vi "Get VS Amplitude String.vi"(10 "text":string, 11 "index":i32) -> (2 "text out":string, 3 "function return":u32)   [LabVIEW 2018, in "Copy of Andor SDK.lvlib"]
doc: "EXPNETTYPE unsigned int WINAPI GetVSAmplitudeString(int index, char * text);"
uses:
  Copy of Andor SDK.lvlib
  <userlib>/Andor SDK/ATMCD32D.dll
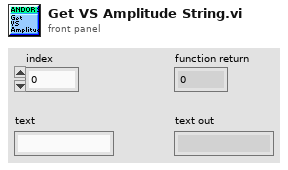
[diagram p1: front panel]
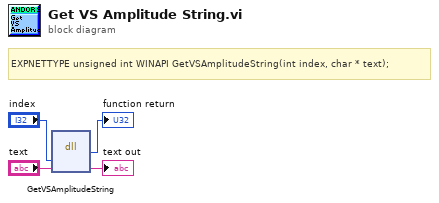
[diagram p0: block diagram]
diagram:
  # "EXPNETTYPE unsigned int WINAPI GetVSAmplitudeString(int index, char * text);"
  n1 = dll-call lib="C:/Program Files (x86)/National Instruments/LabVIEW 2018/user.lib/Andor SDK/ATMCD32D.*" fn="GetVSAmplitudeString"("index"="index", "text"="text") -> (→"function return":u32, "text"=→"text out":string)  [unwired: 4 in, 2 out]
